vi "Mapping Merge Real Positions v10.2.1.vi"(0 "Live Data In":dbl[][](array[numeric]), 5 "X in (1D)":dbl[](array[numeric]), 7 "Y in (1D)":dbl[](array[numeric]), 9 "Step Size":dbl=1.0 caption="Step (µm)" min=0.1 max=30.0 step=0.1 format="%.1f") -> (4 "Live Data Out":dbl[][](array[numeric]))   [LabVIEW 2010]
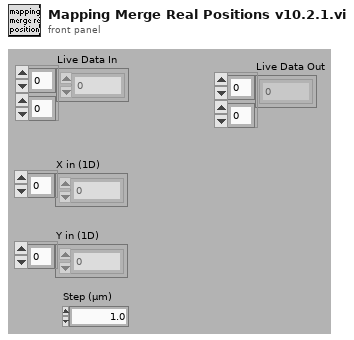
[diagram p1: front panel]
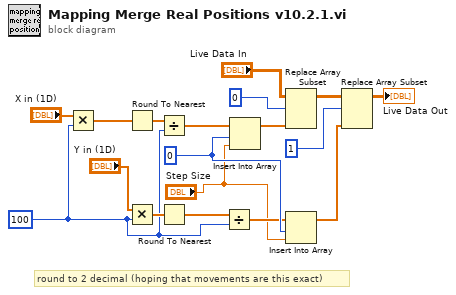
[diagram p0: block diagram]
diagram:
  w4 = i16 100 ("y")
  w18 = 0 ("index")
  # "round to 2 decimal (hoping that movements are this exact)"
  n1 = Multiply(x="X in (1D)", y=w4) -> (x*y=w8:dbl[])
  n2 = Round To Nearest(number=w8) -> (nearest integer value=w5:dbl[])
  n3 = Multiply(x="Y in (1D)", y=w4) -> (x*y=w7:dbl[])
  n4 = Divide(x=w5, y=w4) -> (x/y=w3:dbl[])
  n5 = Round To Nearest(number=w7) -> (nearest integer value=w6:dbl[])
  n6 = Divide(x=w6, y=w4) -> (x/y=w2:dbl[])
  n7 = Insert Into Array(array=w3, index=w18, new element="Step Size") -> (w12:dbl[])
  n8 = Replace Array Subset(array="Live Data In", new element=w12, index (row)=0) -> (w16:dbl[][])  [unwired: 1 in]
  n9 = Insert Into Array(array=w2, index=w18, new element="Step Size") -> (w11:dbl[])
  n10 = Replace Array Subset(array=w16, new element=w11, index (row)=1) -> (→"Live Data Out":dbl[][])  [unwired: 1 in]
